vi "Remove all sections.vi"(11 "info data":string) -> (3 "info data out":string)   [LabVIEW 2020, in "infolib.lvlib"]
doc: "Remove all sections and returns the rest. Contain infinite loop, but every iteration something should be removed, so the loop should always end."
uses:
  infolib.lvlib
  <vilib>/regexp/Match Regular Expression.xnode
panel:
  # "testing string:"
  # "test1\ntest2\n#startsection:: 1\nAAA\n#startsection:: 2\nBBB\n\t  \t#endsection:: 2\nCCC\n#endsection:: 1\ntest3\ntest4\n#startsection:: X\nDDD\n#endsection:: X\ntest5"
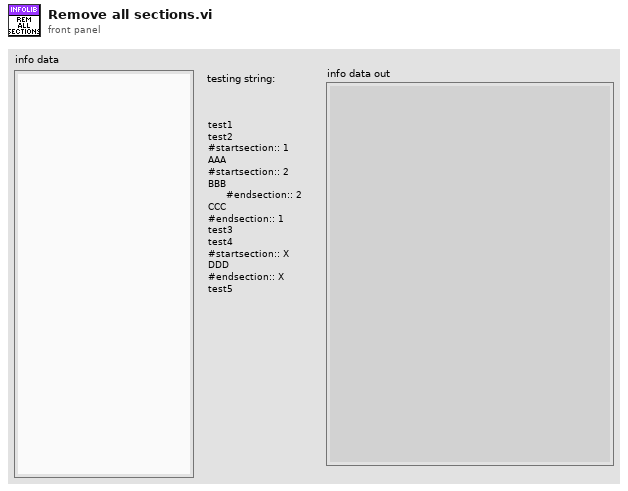
[diagram p1: front panel]
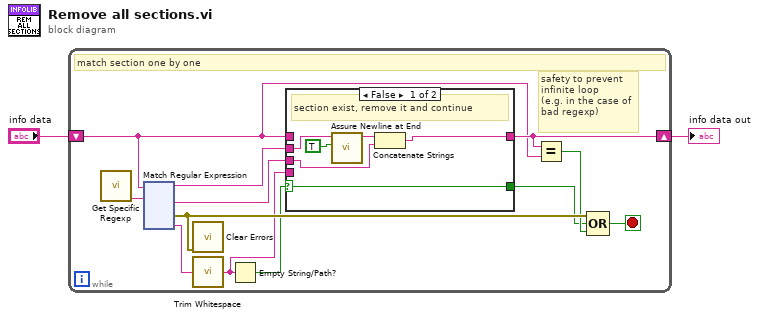
[diagram p0: block diagram]
diagram:
  n1 = while {
    shift-right: [w10] -> w1
    shift-left: "info data" -> [w9]
    stop <- w14 stop-if-true
    # "safety to prevent\ninfinite loop\n(e.g. in the case of\nbad regexp)"
    # "match section one by one"
    n2 = call "Get Specific Regexp.vi"() -> ("Any Section"=w5:string)  [unwired: 8 in, 3 out]
    n3 = xnode "Match Regular Expression"("input string"=w9, "regular expression"=w5) -> ("before match"=w3:string, "after match"=w4:string, "error out"=w13:errorcluster, "submatch 1"=w12:string)  [unwired: 4 in, 2 out]
    n4 = call <vilib>:"Clear Errors.vi"("error in (no error)"=w13) -> ()  [unwired: 5 in, 2 out]
    n5 = call <vilib>:"Trim Whitespace.vi"("string"=w12) -> ("trimmed string"=w11:string)  [unwired: 1 in]
    n6 = Empty String/Path?(string/path=w11) -> (empty?=w7:bool)
    n7 = case shown="False" w7 {
      selector: w7 -> [w15 w21]
      tunnel: w11 -> [_ _]
      tunnel: w9 -> [_ w22]
      tunnel: [w19 w22] -> w10
      tunnel: [w15 w21] -> w6
      tunnel: w4 -> [w16 _]
      tunnel: w3 -> [w17 _]
      frame False {
        # "section exist, remove it and continue"
        n8 = call "Assure Newline at End.vi"("Set End Of Line (F)"=TRUE, "string"=w17) -> ("string out"=w20:string)  [unwired: 9 in]
        n9 = Concatenate Strings(w20, w16) -> (w19:string)
      }
      frame True {
        # "no section, quit"
      }
    }
    n10 = Equal?(x=w10, y=w9) -> (x = y?=w8:bool)
    n11 = Compound Arithmetic op=OR(w13, w6, w8) -> (w14:bool)
  }
  "info data out" <- w1
